vi "GetStatTdmConfig.vi"(0 "storage refnum (file)":refnum<k20>, 1 "error in":errorcluster) -> (2 "storage refnum (file) out":refnum<k20>, 3 "Impedance":dbl, 4 "Voltage Range":dbl, 5 "error out":errorcluster)   [LabVIEW 2014]
uses:
  <vilib>/Platform/storage/lvStorage.llb/_queryPropPoly.vi
  <vilib>/Platform/storage/lvStorage.llb/_queryPropString.vi
  <vilib>/Platform/storage/lvStorage.llb/_queryGenericObjects.vi
  <vilib>/Platform/storage/lvStorage.llb/_loadAllDdt.vi
  <vilib>/Platform/storage/lvStorage.llb/xStorage/xStorageSupp/ErrorOut.vi
  <vilib>/Platform/storage/lvStorage.llb/xStorage/Read Data/Read Data.xnode
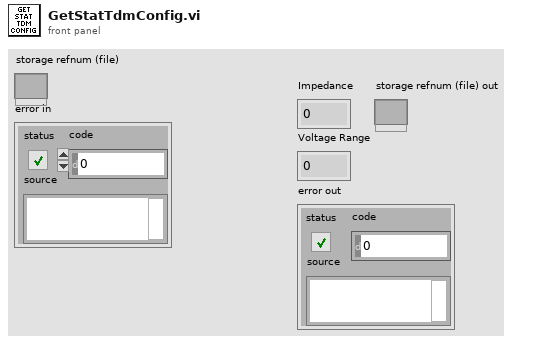
[diagram p1: front panel]
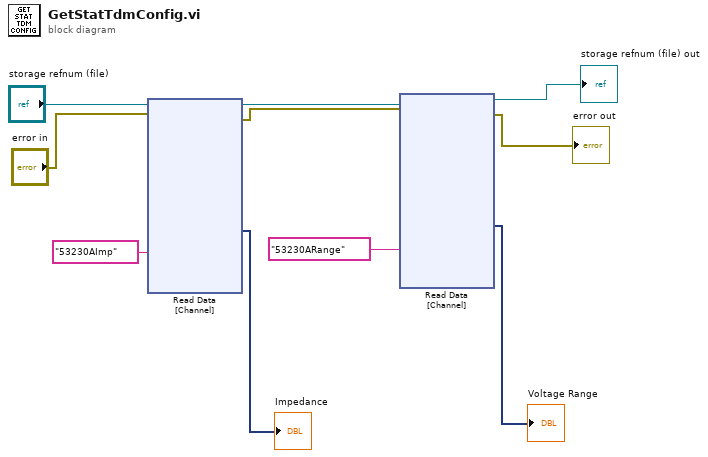
[diagram p0: block diagram]
diagram:
  n1 = xnode "Read Data\n[Channel]"("Name"="53230AImp", "storage refnum (file)"="storage refnum (file)", "error in"="error in") -> ("Signal"=→"Impedance":dynamicdata, "storage refnum (file) out"=w8:refnum<k20>, "error out"=w7:errorcluster)  [unwired: 3 in, 1 out]
  n2 = xnode "Read Data\n[Channel]"("Name"="53230ARange", "storage refnum (file)"=w8, "error in"=w7) -> ("Signal"=→"Voltage Range":dynamicdata, "storage refnum (file) out"=→"storage refnum (file) out":refnum<k20>, "error out"=→"error out":errorcluster)  [unwired: 3 in, 1 out]
